vi "playMp4.vi"(8 "error in (no error)":errorcluster, 10 "playMp4":string, 11 "Mp4Player in":refnum<class "Mp4Player.lvclass">) -> (0 "error out":errorcluster, 3 "Mp4Player out":refnum<class "Mp4Player.lvclass">)   [LabVIEW 2017, in "Mp4Player.lvclass"]
uses:
  Mp4Player.lvclass
  ConsoleOut/Print Options.ctl
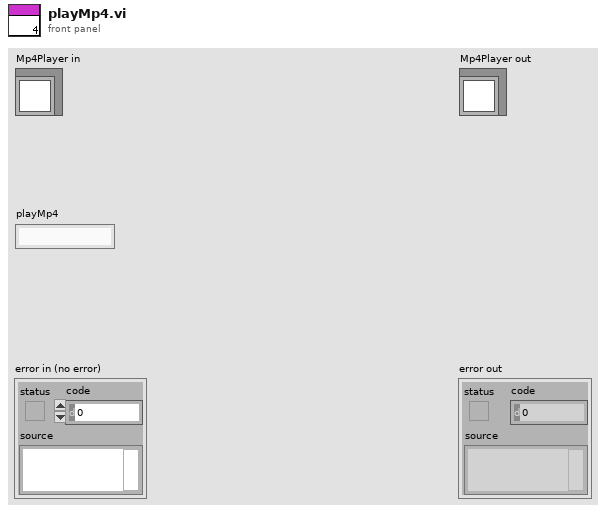
[diagram p1: front panel]
types:
  T1 = typedef "Print Options.ctl" = enum16{"Create", "Get Reference", "Print", "Print Header", "Close"}
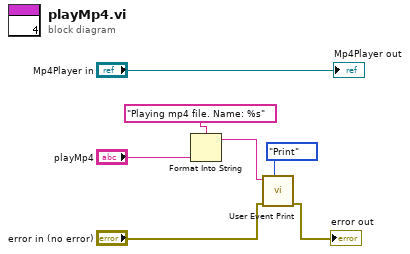
[diagram p0: block diagram]
diagram:
  n1 = Format Into String(format string="Playing mp4 file. Name: %s", "playMp4") -> (resulting string=w4:string)  [unwired: 2 in, 1 out]
  n2 = call "User Event Print.vi"("Options"=Print_Options."Print", "error in (no error)"="error in (no error)", "String to Print"=w4) -> ("error out"=→"error out":errorcluster)  [unwired: 7 in, 1 out]
  "Mp4Player out" <- "Mp4Player in"
